vi "测量流程.vi"(11 "控制命令":T1(ring)) -> ()   [LabVIEW 2016, in "斯坦道氨氮.lvlib"]
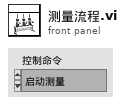
[diagram p1: front panel]
types:
  T1 = enum16{"启动测量", "标样核查", "零点核查", "跨度核查", "空白测试", "平行样测试", "加标回收", "空白校准", "标样校准", "初始化（清洗）", "停止测试", "仪器重启", "校时", "模式设置", "测量间隔设置"}
  T2 = cluster{"站号":u16, "量程切换":enum32{"H", "L", "AUTO"}, "控制命令":enum16{"启动测量", "标样核查", "零点核查", "跨度核查", "空白测试", "平行样测试", "加标回收", "空白校准", "标样校准", "初始化（清洗）", "停止测试", "仪器重启", "校时", "模式设置", "测量间隔设置"}, "模式设置":enum16{"待机", "连续模式", "周期模式", "定点模式", "受控模式", "手动模式"}, "测量间隔":u16}
  T3 = cluster{"时间标识":timestamp, "设备":string, "日志信息":string, "流程参数":string}
  T4 = enum16{"空闲", "水样测试", "标样核查", "零点核查", "跨度核查", "空白测试", "平行样测试", "加标回收", "空白校准", "标样校准", "初始化（清洗）"}
  T5 = cluster{"系统时间":timestamp, "工作状态":enum16{"空闲", "水样测试", "标样核查", "零点核查", "跨度核查", "空白测试", "平行样测试", "加标回收", "空白校准", "标样校准", "初始化（清洗）"}, "测量模式":enum16{"待机", "连续模式", "周期模式", "定点模式", "受控模式", "手动模式"}, "告警代码":u16, "故障代码":u16, "日志代码":u16, "软件版本":u16, "F0":sgl, "F1":sgl, "F2":sgl, "F3":sgl, "T":sgl, "H":sgl, "id":u16, "flowid":u16, "量程":u16, "总磷控温温度1":sgl, "营养盐控温温度2":sgl, "ADC":sgl}
  T6 = cluster{"水样测试量程模式":enum16{"H", "L", "AUTO"}, "空白核查量程模式":enum16{"H", "L", "AUTO"}, "跨度核查量程模式":enum16{"H", "L", "AUTO"}, "加标回收量程模式":enum16{"H", "L", "AUTO"}}
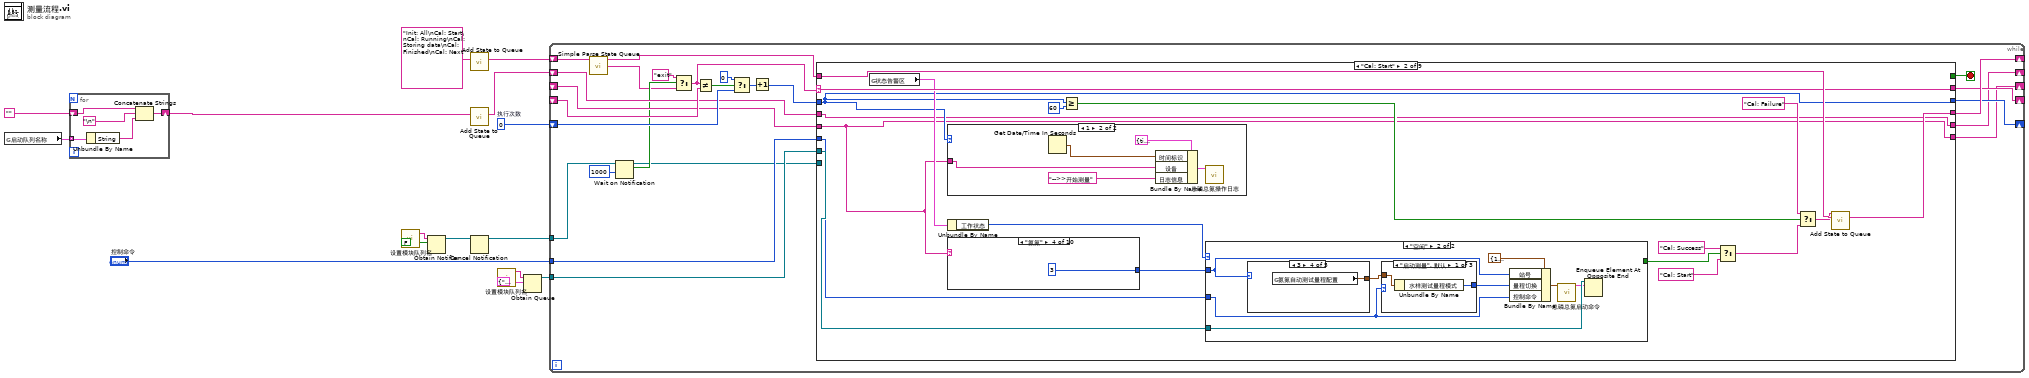
[diagram p0: block diagram]
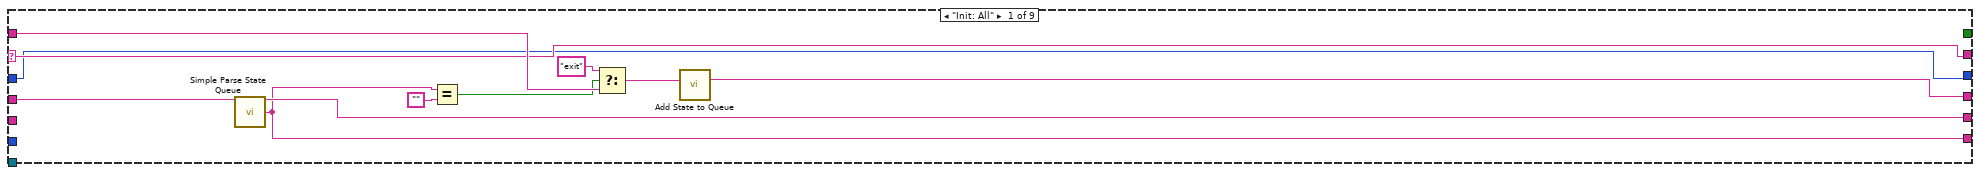
[diagram p2: hidden frame]
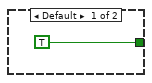
[diagram p3: hidden frame]
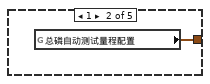
[diagram p5: hidden frame]
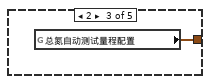
[diagram p6: hidden frame]
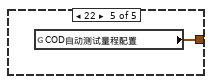
[diagram p7: hidden frame]
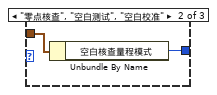
[diagram p8: hidden frame]
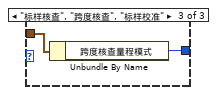
[diagram p9: hidden frame]
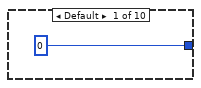
[diagram p10: hidden frame]
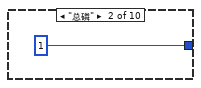
[diagram p11: hidden frame]
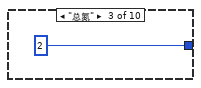
[diagram p12: hidden frame]
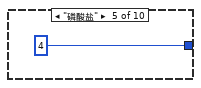
[diagram p13: hidden frame]
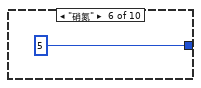
[diagram p14: hidden frame]
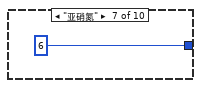
[diagram p15: hidden frame]
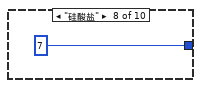
[diagram p16: hidden frame]
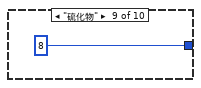
[diagram p17: hidden frame]
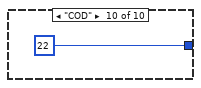
[diagram p18: hidden frame]
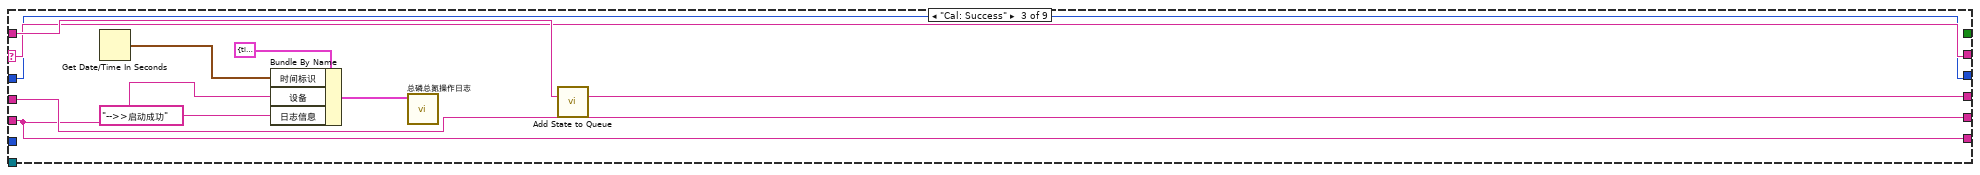
[diagram p20: hidden frame]
diagram:
  w9 = 0  # 执行次数
  n1 = global read "VAR总磷总氮全局变量.vi" "启动队列名称"() -> (w1:cluster{"String":string, "Value":u16}[])
  n2 = for {
    shift-right: [w19] -> w2
    shift-left: "" -> [w20]
    tunnel: w1 -> [w18] mode=indexing
    n3 = Unbundle By Name(w18) -> ("String"=w17:string)
    n4 = Concatenate Strings(w20, "\n", w17) -> (w19:string)
  }
  n5 = call "设置模块队列名.vi"() -> ("Msg"=w6:string)  [unwired: 5 in]
  n6 = Obtain Notifier(name (unnamed)=w6, notification data type=FALSE) -> (notifier out=w14:refnum<notifier>)  [unwired: 2 in, 2 out]
  n7 = call "Add State to Queue.vi"("State(s) In (\"\")"="Init: All\nCal: Start\nCal: Running\nCal: Storing data\nCal: Finished\nCal: Next" ("State(s) In (\"\")")) -> ("States Out"=w12:string)  [unwired: 14 in]
  n8 = call "Add State to Queue.vi"("State(s) In (\"\")"=w2) -> ("States Out"=w7:string)  [unwired: 14 in]
  n9 = Cancel Notification(0:w14) -> (8:w4:refnum<notifier>)  [unwired: 1 in, 2 out]
  n10 = call "设置模块队列名.vi"() -> ("Msg"=w5:string)  [unwired: 5 in]
  n11 = Obtain Queue(name (unnamed)=w5, element data type=cluster{"命令":string, "data":variant} {"命令"="", "data"=variant}) -> (queue out=w10:refnum<queue>)  [unwired: 3 in, 2 out]
  n12 = while {
    tunnel: w10 -> [w43]
    shift-right: [w42] -> _
    shift-left: w12 -> [w45]
    shift-right: [w35] -> _
    shift-left: w9 -> [w38]
    shift-right: [w41] -> _
    shift-left: _ -> [w40]
    tunnel: "控制命令" -> [w33]
    shift-right: [w29] -> _
    shift-left: w7 -> [w31]
    shift-right: [w30] -> _
    shift-left: _ -> [w28]
    tunnel: w4 -> [w26]
    stop <- w32 stop-if-true
    n13 = call "Simple Parse State Queue.vi"("State Queue"=w45) -> ("Remain States"=w44:string, "Next State"=w23:string)  [unwired: 13 in]
    n14 = Wait on Notification(notifier=w26, timeout in ms (-1)=1000 ("超时毫秒(-1)")) -> (notifier out=w21:refnum<notifier>, notification=w25:bool)  [unwired: 2 in, 2 out]
    n15 = Select(t="exit", s=w25, f=w23) -> (s? t:f=w22:string)
    n16 = Not Equal?(x=w22, y=w40) -> (x != y?=w39:bool)
    n17 = Select(t=0, s=w39, f=w38) -> (s? t:f=w36:i32)
    n18 = Increment(x=w36) -> (x+1=w34:i32)
    n19 = case shown="\"Cal: Start\"" w22 {
      selector: w22 -> [w52 w73 w113 w128 w134 w148 w164 w175 w182]
      tunnel: w44 -> [w54 w75 w115 _ w145 w153 w166 _ w183]
      tunnel: w43 -> [_ w71 _ _ _ _ _ _ w178]
      tunnel: [w56 w74 w114 w129 w144 w152 w165 "Init: All\nCal: Start\nCal: Running\nCal: Storing data\nCal: Finished\nCal: Next" ("State(s) In (\"\")") w183] -> w42
      tunnel: [w52 w73 w113 w128 w134 w148 w164 w175 w182] -> w41
      tunnel: [w51 w68 w112 w127 w137 w151 w162 w174 w181] -> w35
      tunnel: w34 -> [w51 w68 w112 w127 w137 w151 w162 w174 w181]
      tunnel: w33 -> [_ w70 _ _ _ _ _ _ _]
      tunnel: [_ _ _ _ _ _ _ _ TRUE] -> w32
      tunnel: w31 -> [w50 w57 w111 w121 w131 w155 w163 w173 w180]
      tunnel: [w48 w58 w110 w120 w130 w154 w161 w172 w179] -> w30
      tunnel: [w49 w57 w111 w121 w131 w155 w163 w173 w180] -> w29
      tunnel: w28 -> [_ w58 w110 w120 w130 w154 w161 w172 w179]
      tunnel: w21 -> [_ _ _ _ _ _ _ _ w177]
      frame "Init: All" {
        n20 = call "Simple Parse State Queue.vi"("State Queue"=w50) -> ("Remain States"=w49:string, "Next State"=w48:string)  [unwired: 13 in]
        n21 = Equal?(x=w48, y="") -> (x = y?=w46:bool)
        n22 = Select(t="exit", s=w46, f=w54) -> (s? t:f=w53:string)
        n23 = call "Add State to Queue.vi"("State(s) In (\"\")"=w53) -> ("States Out"=w56:string)  [unwired: 14 in]
      }
      frame "Cal: Start" {
        n24 = global read "VAR总磷总氮全局变量.vi" "状态告警区"() -> (w72:T5)
        n25 = case shown="1" w68 {
          tunnel: w58 -> [_ w105]
          frame 0, Default {
          }
          frame 1 {
            n26 = Get Date/Time In Seconds() -> (seconds since 1Jan1904=w109:timestamp)
            n27 = Bundle By Name(cluster=T3 {"时间标识"=timestamp(0 s since 1904-01-01), "设备"="", "日志信息"="", "流程参数"=""} ("data in"), "时间标识"=w109, "设备"=w105, "日志信息"="-->>开始测量") -> (w108:T3)
            n28 = call "总磷总氮操作日志.vi"("data in"=w108) -> ()  [unwired: 11 in]
          }
        }
        n29 = Unbundle By Name(w72) -> ("工作状态"=w59:T4)
        n30 = case shown="\"氨氮\"" w58 {
          tunnel: [0 1 2 3 4 5 6 7 8 22] -> w69
          frame Default {
          }
          frame "总磷" {
          }
          frame "总氮" {
          }
          frame "氨氮" {
          }
          frame "磷酸盐" {
          }
          frame "硝氮" {
          }
          frame "亚硝氮" {
          }
          frame "硅酸盐" {
          }
          frame "硫化物" {
          }
          frame "COD" {
          }
        }
        n31 = Greater Or Equal?(x=w68, y=60) -> (x >= y?=w66:bool)
        n32 = case shown="\"空闲\"" w59 {
          tunnel: w70 -> [_ w80]
          tunnel: w71 -> [_ w83]
          tunnel: [TRUE _] -> w63
          tunnel: w69 -> [_ w78]
          frame Default {
          }
          frame "空闲" {
            n33 = case shown="3" w78 {
              tunnel: [_ w85 w86 w87 w88] -> w79
              frame 0, Default {
              }
              frame 1 {
                n34 = global read "总磷总氮断电保存全局变量.vi" "总磷自动测试量程配置"() -> (w85:T6)
              }
              frame 2 {
                n35 = global read "总磷总氮断电保存全局变量.vi" "总氮自动测试量程配置"() -> (w86:T6)
              }
              frame 3 {
                n36 = global read "总磷总氮断电保存全局变量.vi" "氨氮自动测试量程配置"() -> (w87:T6)
              }
              frame 22 {
                n37 = global read "总磷总氮断电保存全局变量.vi" "COD自动测试量程配置"() -> (w88:T6)
              }
            }
            n38 = case shown="\"启动测量\", 默认" w80 {
              tunnel: w79 -> [w90 w92 w94]
              tunnel: [w89 w91 w93] -> w84
              frame "启动测量", Default {
                n39 = Unbundle By Name(w90) -> ("水样测试量程模式"=w89:enum16{"H", "L", "AUTO"})
              }
              frame "零点核查", "空白测试", "空白校准" {
                n40 = Unbundle By Name(w92) -> ("空白核查量程模式"=w91:enum16{"H", "L", "AUTO"})
              }
              frame "标样核查", "跨度核查", "标样校准" {
                n41 = Unbundle By Name(w94) -> ("跨度核查量程模式"=w93:enum16{"H", "L", "AUTO"})
              }
            }
            n42 = Bundle By Name(cluster=T2 {"站号"=1, "量程切换"=enum."AUTO", "控制命令"=enum."启动测量", "模式设置"=enum."待机", "测量间隔"=0} ("参数"), "站号"=w78, "量程切换"=w84, "控制命令"=w80) -> (w81:T2)
            n43 = call "总磷总氮启动命令.vi"("参数"=w81) -> ("启动命令"=w77:cluster{"命令":string, "data":variant})  [unwired: 10 in]
            n44 = Enqueue Element At Opposite End(queue=w83, element=w77) -> ()  [unwired: 2 in, 3 out]
          }
        }
        n45 = Select(t="Cal: Success" ("State(s) In (\"\")"), s=w63, f="Cal: Start" ("State(s) In (\"\")")) -> (s? t:f=w61:string)
        n46 = Select(t="Cal: Failure" ("State(s) In (\"\")"), s=w66, f=w61) -> (s? t:f=w64:string)
        n47 = call "Add State to Queue.vi"("State(s) In Front (\"\")"=w64, "State(s) In (\"\")"=w75) -> ("States Out"=w74:string)  [unwired: 13 in]
      }
      frame "Cal: Success" {
        n48 = Get Date/Time In Seconds() -> (seconds since 1Jan1904=w118:timestamp)
        n49 = Bundle By Name(cluster=T3 {"时间标识"=timestamp(0 s since 1904-01-01), "设备"="", "日志信息"="", "流程参数"=""} ("data in"), "时间标识"=w118, "设备"=w110, "日志信息"="-->>启动成功") -> (w117:T3)
        n50 = call "总磷总氮操作日志.vi"("data in"=w117) -> ()  [unwired: 11 in]
        n51 = call "Add State to Queue.vi"("State(s) In (\"\")"=w115) -> ("States Out"=w114:string)  [unwired: 14 in]
      }
      frame "Cal: Failure" {
        n52 = Get Date/Time In Seconds() -> (seconds since 1Jan1904=w125:timestamp)
        n53 = Bundle By Name(cluster=T3 {"时间标识"=timestamp(0 s since 1904-01-01), "设备"="", "日志信息"="", "流程参数"=""} ("data in"), "时间标识"=w125, "设备"=w120, "日志信息"="-->>启动失败") -> (w124:T3)
        n54 = call "总磷总氮操作日志.vi"("data in"=w124) -> ()  [unwired: 11 in]
        n55 = call "Add State to Queue.vi"("State(s) In (\"\")"="exit" ("State(s) In (\"\")")) -> ("States Out"=w129:string)  [unwired: 14 in]
      }
      frame "Cal: Running" {
        n56 = global read "VAR总磷总氮全局变量.vi" "状态告警区"() -> (w141:T5)
        n57 = Unbundle By Name(w141) -> ("工作状态"=w142:T4)
        n58 = Less Or Equal?(x=w137, y=7200) -> (x <= y?=w135:bool)
        n59 = Select(t=w134, s=w135, f="exit") -> (s? t:f=w133:string)
        n60 = Equal?(x=w142, y=T4."空闲") -> (x = y?=w140:bool)
        n61 = Select(t="", s=w140, f=w133) -> (s? t:f=w138:string)
        n62 = call "Add State to Queue.vi"("State(s) In Front (\"\")"=w138, "State(s) In (\"\")"=w145) -> ("States Out"=w144:string)  [unwired: 13 in]
      }
      frame "Cal: Storing data" {
        n63 = case shown="1" w151 {
          tunnel: w154 -> [_ w156]
          frame 0, Default {
          }
          frame 1 {
            n64 = Get Date/Time In Seconds() -> (seconds since 1Jan1904=w160:timestamp)
            n65 = Bundle By Name(cluster=T3 {"时间标识"=timestamp(0 s since 1904-01-01), "设备"="", "日志信息"="", "流程参数"=""} ("data in"), "时间标识"=w160, "设备"=w156, "日志信息"="-->>存储数据") -> (w159:T3)
            n66 = call "总磷总氮操作日志.vi"("data in"=w159) -> ()  [unwired: 11 in]
          }
        }
        n67 = Less Or Equal?(x=w151, y=10) -> (x <= y?=w149:bool)
        n68 = Select(t=w148, s=w149, f="") -> (s? t:f=w146:string)
        n69 = call "Add State to Queue.vi"("State(s) In Front (\"\")"=w146, "State(s) In (\"\")"=w153) -> ("States Out"=w152:string)  [unwired: 13 in]
      }
      frame "Cal: Finished" {
        n70 = call "Add State to Queue.vi"("State(s) In (\"\")"=w166) -> ("States Out"=w165:string)  [unwired: 14 in]
        n71 = case shown="1" w162 {
          tunnel: w161 -> [_ w167]
          frame 0, Default {
          }
          frame 1 {
            n72 = Get Date/Time In Seconds() -> (seconds since 1Jan1904=w171:timestamp)
            n73 = Bundle By Name(cluster=T3 {"时间标识"=timestamp(0 s since 1904-01-01), "设备"="", "日志信息"="", "流程参数"=""} ("data in"), "时间标识"=w171, "设备"=w167, "日志信息"="-->>测量结束") -> (w170:T3)
            n74 = call "总磷总氮操作日志.vi"("data in"=w170) -> ()  [unwired: 11 in]
          }
        }
      }
      frame "Cal: Next" {
      }
      frame "exit", Default {
        n75 = Release Queue(queue=w178) -> ()  [unwired: 2 in, 3 out]
        n76 = Release Notifier(notifier=w177) -> ()  [unwired: 2 in, 3 out]
      }
    }
  }
